vi "camera_initialise_start_settings_AVT_Pike_F032B.vi"(6 "Gain (0-630)":u32=500, 8 "error in":errorcluster, 9 "Video Mode":u32=2, 10 "Shutter time (ms)":dbl=100.0, 11 "Camera In":T1="cam0") -> (0 "Fehler (Ausgang)":errorcluster, 3 "Camera Out":T1)   [LabVIEW 2009]
uses:
  <vilib>/userDefined/High Color/IMAQdx.ctl
  <vilib>/vision/driver/NI_Vision_Acquisition_Software.lvlib
  C:/Program Files/National Instruments/LabVIEW 2009/resource/objmgr/imaqdx.rc
panel:
  in  "Y Offset (px)":u32
  in  "X Offset (px)":u32
  in  "Image Height (px)":u32=480
  in  "Image Width (px)":u32=640
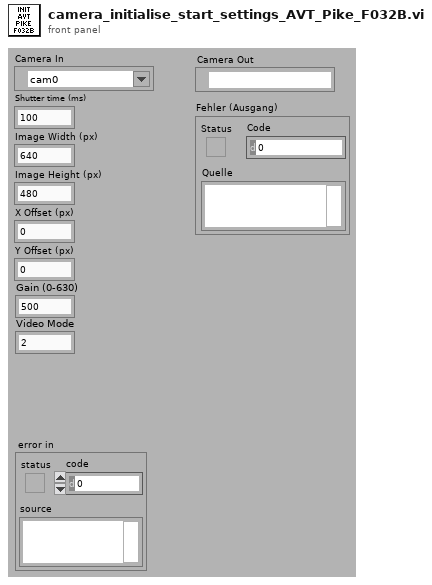
[diagram p1: front panel]
types:
  T1 = typedef "IMAQdx.ctl" = refnum<k21>
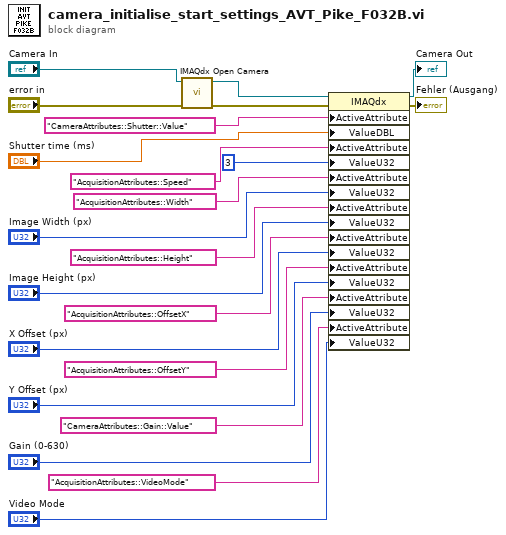
[diagram p0: block diagram]
diagram:
  n1 = call <vilib>:"IMAQdx Open Camera.vi"("error in"="error in", "Session In"="Camera In") -> ("error out"=w20:errorcluster, "Session Out"=w21:T1)  [unwired: 8 in]
  n2 = property class="IMAQdx"(reference=w21, error in=w20, "ActiveAttribute"="CameraAttributes::Shutter::Value", "ValueDBL"="Shutter time (ms)", "ActiveAttribute"="AcquisitionAttributes::Speed", "ValueU32"=u32 3, "ActiveAttribute"="AcquisitionAttributes::Width", "ValueU32"="Image Width (px)", "ActiveAttribute"="AcquisitionAttributes::Height", "ValueU32"="Image Height (px)", "ActiveAttribute"="AcquisitionAttributes::OffsetX", "ValueU32"="X Offset (px)", "ActiveAttribute"="AcquisitionAttributes::OffsetY", "ValueU32"="Y Offset (px)", "ActiveAttribute"="CameraAttributes::Gain::Value", "ValueU32"="Gain (0-630)", "ActiveAttribute"="AcquisitionAttributes::VideoMode", "ValueU32"="Video Mode") -> (reference out=→"Camera Out":T1, error out=→"Fehler (Ausgang)":errorcluster)
